vi "Create.vi"(8 "error in (no error)":errorcluster, 9 "Main Filename":string, 10 "Config Root":path, 11 "Node Name":string) -> (0 "error out":errorcluster, 3 "VolatusConfig out":refnum<class "VolatusConfigManager.lvclass">)   [LabVIEW 2020, in "Volatus.lvlib" / "VolatusConfigManager.lvclass"]
uses:
  VolatusConfigManager.lvclass
  VolatusConfigManager.lvclass/VolatusConfigManager.ctl
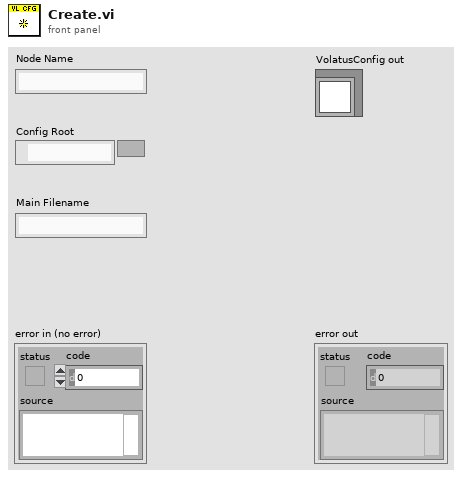
[diagram p1: front panel]
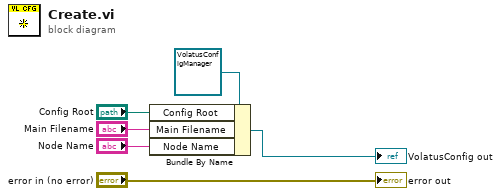
[diagram p0: block diagram]
diagram:
  n1 = Bundle By Name(cluster=refnum<class "VolatusConfigManager.lvclass"> refnum ("VolatusConfig in"), "Config Root"="Config Root", "Main Filename"="Main Filename", "Node Name"="Node Name") -> (→"VolatusConfig out":refnum<class "VolatusConfigManager.lvclass">)
  "error out" <- "error in (no error)"
